vi "Autonomous Independent.vi"   [LabVIEW 2012]
doc: "This VI is called when autonomous begins, and will automatically be terminated when autonomous ends. You can carry out timed or sensor driven robot movement independently without needing to return to the caller."
uses:
  <vilib>/Rock Robotics/WPI/Relay/WPI_RelayValue.ctl
  <vilib>/Rock Robotics/WPI/DriverStation/DriverStationLCD/WPI_DriverStationLCDLCDLine.ctl
  <vilib>/Rock Robotics/WPI/CAN/Jaguar/SubVIs/WPI_CANJaguar_ControlMode.ctl
  <vilib>/Rock Robotics/WPI/CAN/Jaguar/SubVIs/WPI_CANJaguar_PositionReference.ctl
  <vilib>/Rock Robotics/WPI/CAN/Jaguar/SubVIs/WPI_CANJaguar_SpeedReference.ctl
  Robot Global Data.vi
types:
  T1 = typedef "WPI_DriverStationLCDLCDLine.ctl" = enum16{"Main - Line 1", "User - Line 2", "User - Line 3", "User - Line 4", "User - Line 5", "User - Line 6"}
  T2 = typedef "WPI_RelayValue.ctl" = enum16{"Off", "On", "Forward", "Reverse"}
  T3 = typedef "WPI_CANJaguar_ControlMode.ctl" = enum8{"Percent VBus", "Current", "Speed", "Position", "Voltage"}
  T4 = typedef "WPI_MotorControlDeviceRef.ctl" = cluster{"DeviceStatus":errorcluster, "Type":enum16{"PWM", "CAN"}, "PWM":cluster{"Digital Module":T5, "PWM Channel":T6, "DeadBand":T7}, "CAN":cluster{"Device Number":u8, "Control Mode":T3, "Semaphore":T8, "Max Vout":dbl}, "Invert":bool, "TransformRef":T9, "InvTransformRef":T9}
  T5 = typedef "FPGA_TypedefDigitalModule.ctl" = enum16{"Digital Module 1", "Digital Module 2"}
  T6 = typedef "FPGA_DIOPWMChannel.ctl" = enum8{"PWM 1", "PWM 2", "PWM 3", "PWM 4", "PWM 5", "PWM 6", "PWM 7", "PWM 8", "PWM 9", "PWM 10", "Invalid"}
  T7 = typedef "WPI_PWMDeadband.ctl" = cluster{"Name":string, "maxPositivePwm":i32, "minPositivePwm":i32, "centerPwm":i32, "maxNegativePwm":i32, "minNegativePwm":i32, "angularRange":u16}
  T8 = typedef "Semaphore RefNum" = refnum<k1>
  T9 = typedef "WPI_PWMTransform_ConPane.ctl" = refnum<vi>
  T10 = typedef "WPI_RelayDevRef.ctl" = cluster{"DevStatus":errorcluster, "Relay Channel":T11, "Digital Module":T5, "Relay Direction":T12}
  T11 = typedef "FPGA_DIORelayChannel.ctl" = enum8{"Relay 1", "Relay 2", "Relay 3", "Relay 4", "Relay 5", "Relay 6", "Relay 7", "Relay 8", "Invalid"}
  T12 = typedef "WPI_RelayDirection.ctl" = enum16{"Both directions", "Forward only", "Reverse only"}
  T13 = typedef "WPI_CANJaguar_PositionReference.ctl" = u8
  T14 = typedef "WPI_CANJaguar_SpeedReference.ctl" = u8
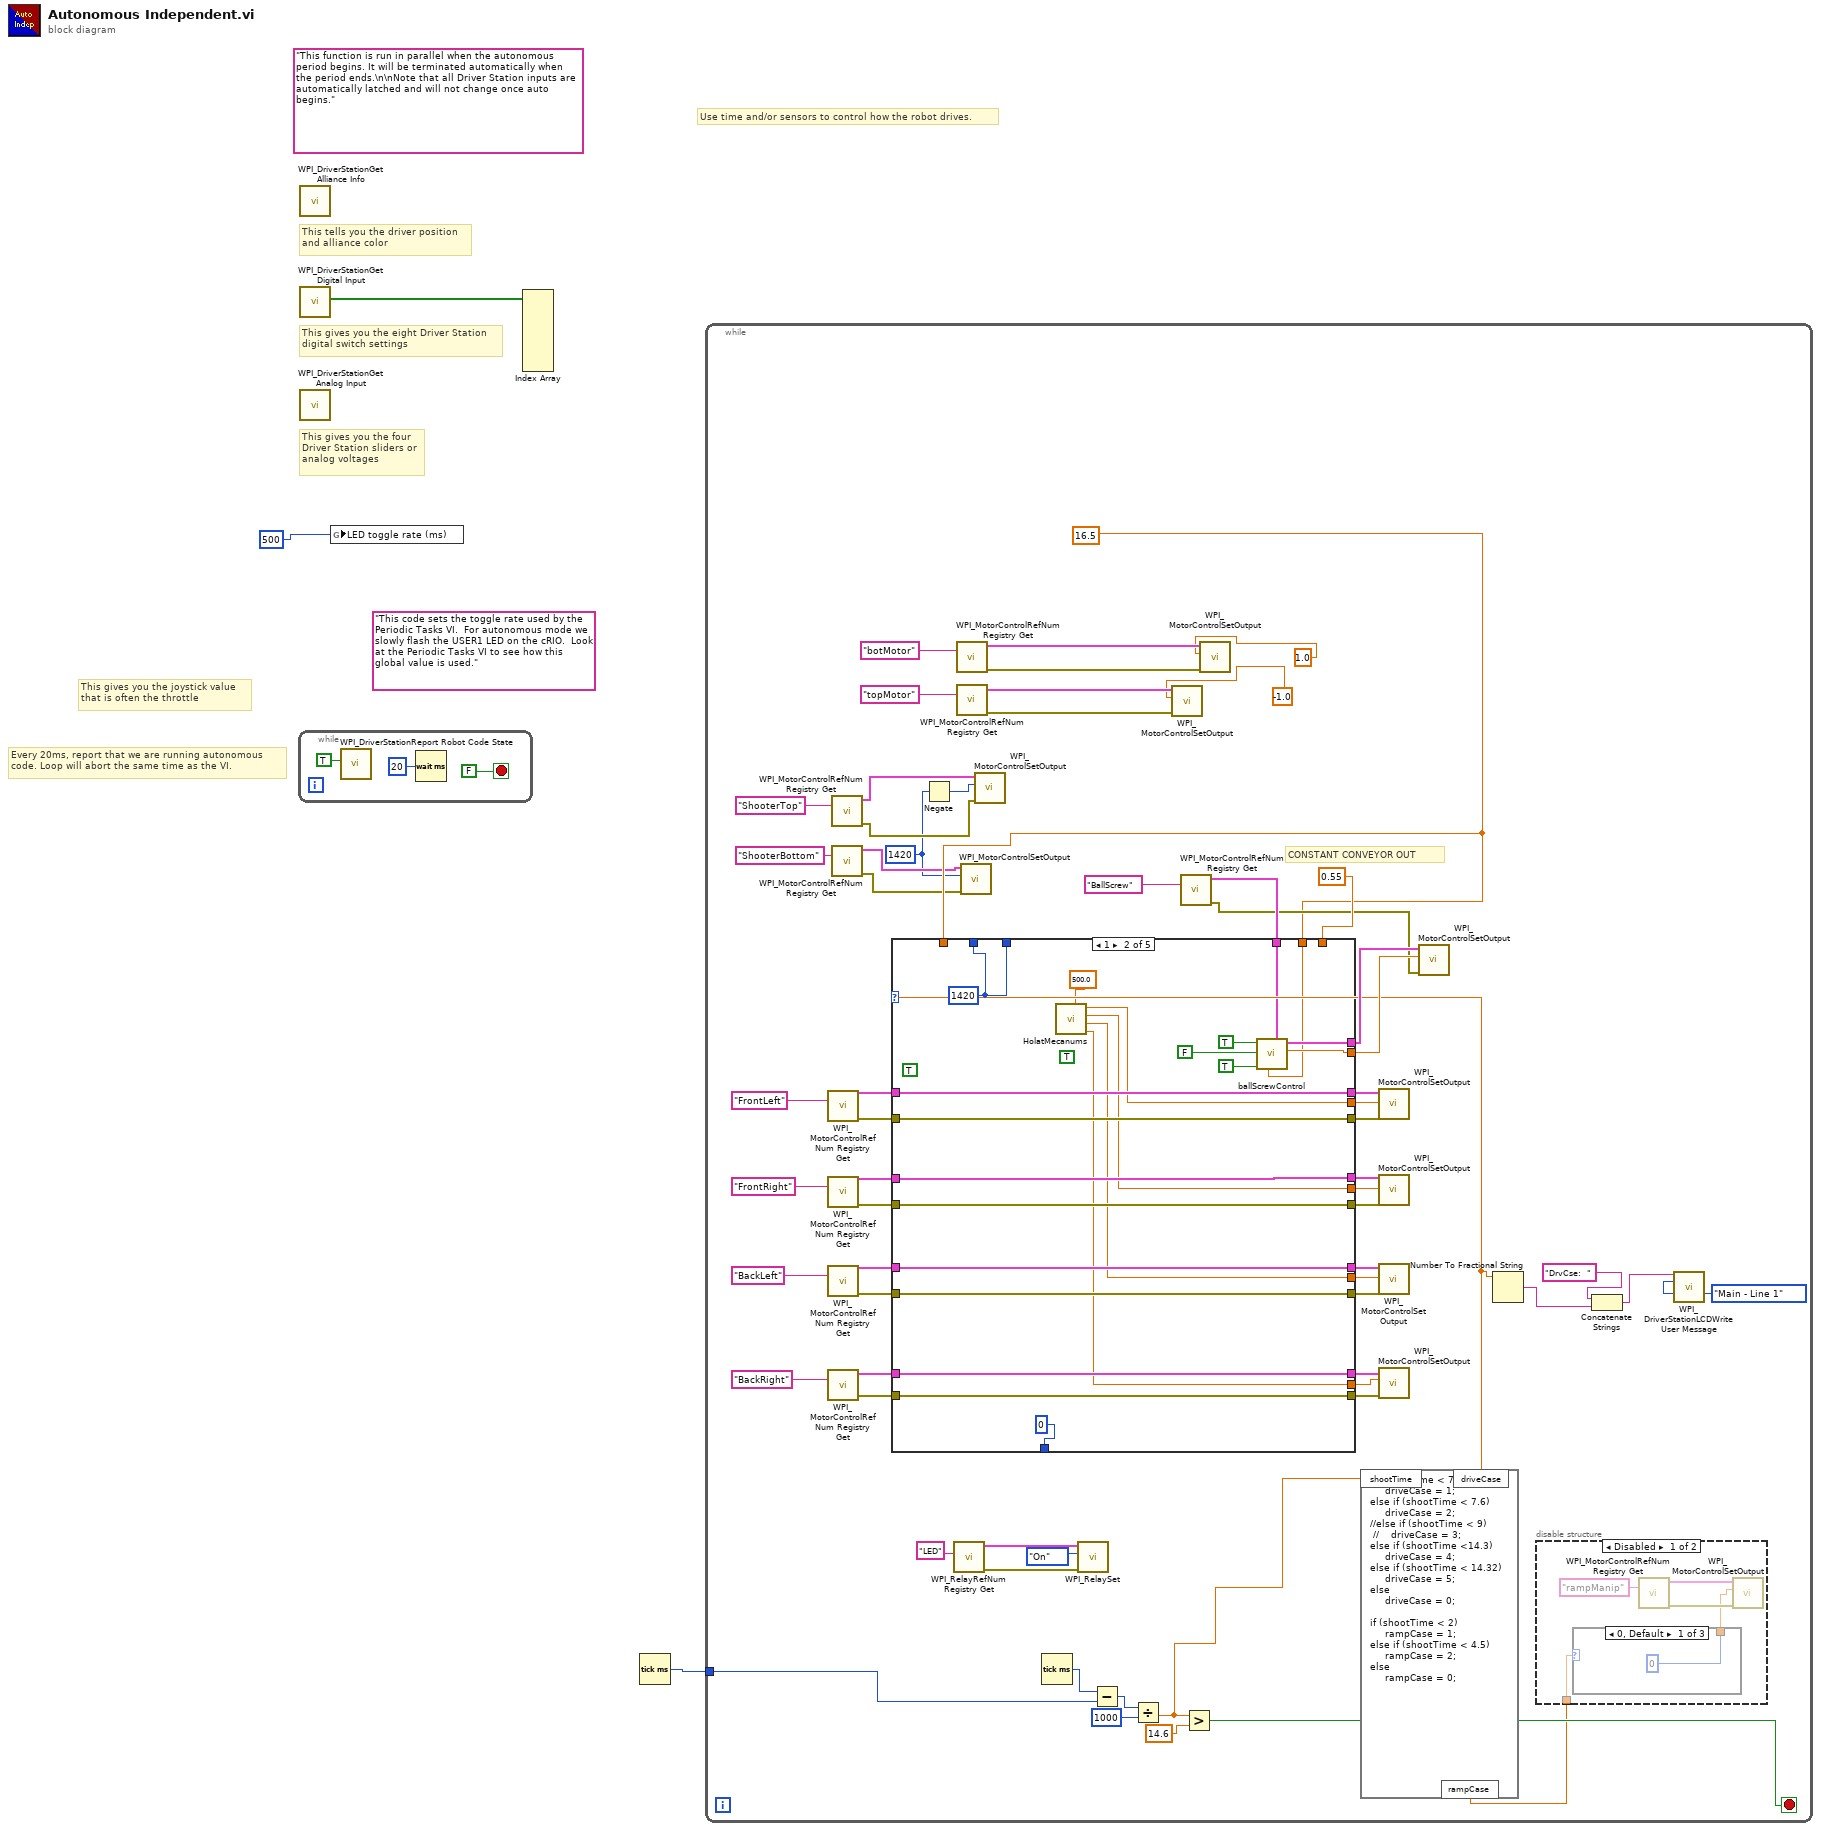
[diagram p0: block diagram]
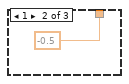
[diagram p2: hidden frame]
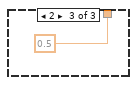
[diagram p3: hidden frame]
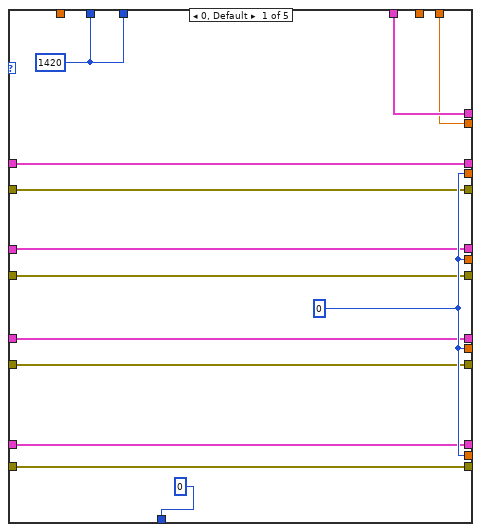
[diagram p5: hidden frame]
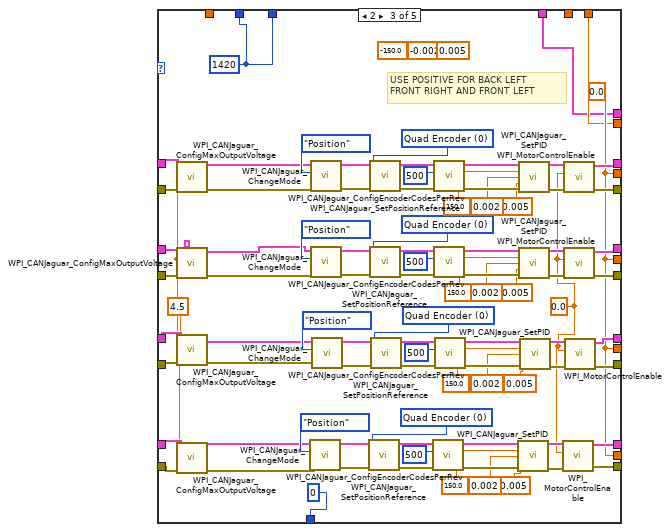
[diagram p6: hidden frame]
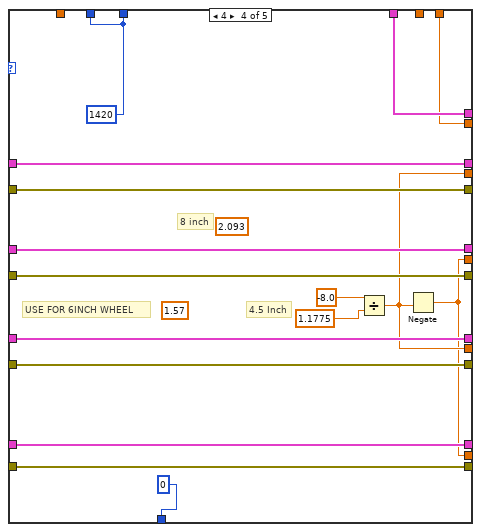
[diagram p7: hidden frame]
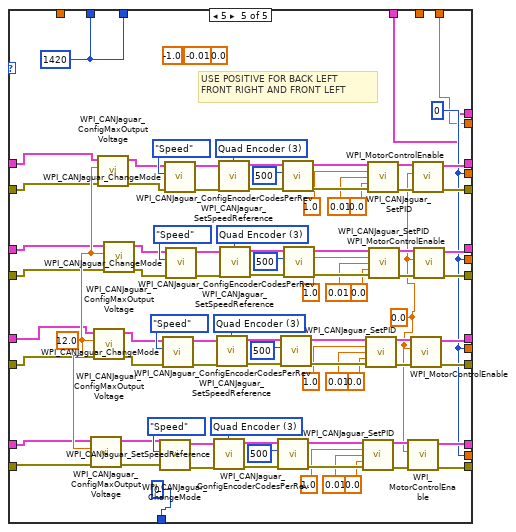
[diagram p8: hidden frame]
diagram:
  (unwired) "This code sets the toggle rate used by the Periodic Tasks VI.  For autonomous mode we slowly flash the USER1 LED on the cRIO.  Look at the Periodic Tasks VI to see how this global value is used."
  (unwired) "This function is run in parallel when the autonomous period begins. It will be terminated automatically when the period ends.\n\nNote that all Driver Station inputs are automatically latched and will not change once auto begins."
  # "Every 20ms, report that we are running autonomous\ncode. Loop will abort the same time as the VI."
  # "This gives you the joystick value\nthat is often the throttle"
  # "Use time and/or sensors to control how the robot drives."
  # "This tells you the driver position\nand alliance color"
  # "This gives you the eight Driver Station\ndigital switch settings"
  # "This gives you the four\nDriver Station sliders or\nanalog voltages"
  n1 = while {
    stop <- FALSE stop-if-true
    n2 = call <vilib>:"WPI_DriverStationReport Robot Code State.vi"("Autonomous"=TRUE) -> ()  [unwired: 10 in, 1 out]
    n3 = Wait (ms)(milliseconds to wait=u32 20) -> ()  [unwired: 1 out]
  }
  n4 = call <vilib>:"WPI_DriverStationGet Alliance Info.vi"() -> ()  [unwired: 12 out]
  n5 = call <vilib>:"WPI_DriverStationGet Digital Input.vi"() -> ("Driver Station Digital Input (1-8)"=w3:bool[])  [unwired: 11 out]
  n6 = call <vilib>:"WPI_DriverStationGet Analog Input.vi"() -> ()  [unwired: 12 out]
  n7 = global write "Robot Global Data.vi" "LED toggle rate (ms)"(u32 500 ("LED ms toggle rate")) -> ()
  n8 = Index Array(array=w3) -> ()  [unwired: 8 in, 8 out]
  n9 = Tick Count (ms)() -> (millisecond timer value=w2:u32)
  n10 = while {
    tunnel: w2 -> [w25]
    stop <- w26 stop-if-true
    w7 = 1420
    w13 = 16.5
    # "CONSTANT CONVEYOR OUT"
    n11 = call <vilib>:"WPI_MotorControlRefNum Registry Get.vi"("refnum name"="FrontLeft") -> ("error out"=w55:errorcluster, "MotorControlDevRef"=w54:T4)  [unwired: 9 in]
    n12 = call <vilib>:"WPI_MotorControlRefNum Registry Get.vi"("refnum name"="FrontRight") -> ("error out"=w57:errorcluster, "MotorControlDevRef"=w56:T4)  [unwired: 9 in]
    n13 = call <vilib>:"WPI_MotorControlRefNum Registry Get.vi"("refnum name"="BackLeft") -> ("error out"=w59:errorcluster, "MotorControlDevRef"=w58:T4)  [unwired: 9 in]
    n14 = call <vilib>:"WPI_MotorControlRefNum Registry Get.vi"("refnum name"="BackRight") -> ("error out"=w60:errorcluster, "MotorControlDevRef"=w61:T4)  [unwired: 9 in]
    n15 = call <vilib>:"WPI_MotorControlRefNum Registry Get.vi"("refnum name"="ShooterTop") -> ("error out"=w10:errorcluster, "MotorControlDevRef"=w11:T4)  [unwired: 9 in]
    n16 = call <vilib>:"WPI_MotorControlRefNum Registry Get.vi"("refnum name"="ShooterBottom") -> ("error out"=w8:errorcluster, "MotorControlDevRef"=w9:T4)  [unwired: 9 in]
    n17 = Negate(x=w7) -> (-x=w12:i32)
    n18 = call <vilib>:"WPI_RelayRefNum Registry Get.vi"("refnum name"="LED") -> ("error out"=w66:errorcluster, "RelayDevRef"=w67:T10)  [unwired: 9 in]
    n19 = call <vilib>:"WPI_MotorControlRefNum Registry Get.vi"("refnum name"="botMotor") -> ("error out"=w51:errorcluster, "MotorControlDevRef"=w52:T4)  [unwired: 9 in]
    n20 = call <vilib>:"WPI_MotorControlRefNum Registry Get.vi"("refnum name"="topMotor") -> ("error out"=w50:errorcluster, "MotorControlDevRef"=w69:T4)  [unwired: 9 in]
    n21 = call <vilib>:"WPI_MotorControlSetOutput.vi"("error in (no error)"=w8, "Output"=w7, "MotorControlDevRef"=w9) -> ()  [unwired: 6 in, 3 out]
    n22 = call <vilib>:"WPI_MotorControlSetOutput.vi"("error in (no error)"=w10, "Output"=w12, "MotorControlDevRef"=w11) -> ()  [unwired: 6 in, 3 out]
    n23 = Tick Count (ms)() -> (millisecond timer value=w46:u32)
    n24 = call <vilib>:"WPI_RelaySet.vi"("error in (no error)"=w66, "RelayValue"=WPI_RelayValue."On", "RelayDevRef"=w67) -> ()  [unwired: 7 in, 2 out]
    n25 = Subtract(x=w46, y=w25) -> (x-y=w45:u32)
    n26 = Divide(x=w45, y=u32 1000) -> (x/y=w27:dbl)
    n27 = call <vilib>:"WPI_MotorControlSetOutput.vi"("error in (no error)"=w50, "Output"=-1.0, "MotorControlDevRef"=w69) -> ()  [unwired: 6 in, 3 out]
    n28 = call <vilib>:"WPI_MotorControlRefNum Registry Get.vi"("refnum name"="BallScrew") -> ("error out"=w20:errorcluster, "MotorControlDevRef"=w24:T4)  [unwired: 9 in]
    n29 = Greater?(x=w27, y=14.6) -> (0:w26:bool)
    n30 = call <vilib>:"WPI_MotorControlSetOutput.vi"("error in (no error)"=w51, "Output"=1.0, "MotorControlDevRef"=w52) -> ()  [unwired: 6 in, 3 out]
    n31 = formula code="if (shootTime < 7.5)\n     driveCase = 1;\nelse if (shootTime < 7.6)\n     driveCase = 2;\n//else if (shootTime < 9)\n //    driveCase = 3;\nelse if (shootTime <14.3)\n     driveCase = 4;\nelse if (shootTime < 14.32)\n     driveCase = 5;\nelse\n     driveCase = 0;\n\nif (shootTime < 2)\n     rampCase = 1;\nelse if (shootTime < 4.5)\n     rampCase = 2;\nelse\n     rampCase = 0;"("shootTime"=w27) -> ("driveCase"=w14:dbl, "rampCase"=w19:dbl)
    n32 = case shown="1" w14 {
      tunnel: [w83 w112 w185 w216 w289] -> w36
      tunnel: w54 -> [w83 w112 w129 w216 w229]
      tunnel: [w85 w111 w170 w214 w273] -> w37
      tunnel: w56 -> [w85 w111 w134 w214 w231]
      tunnel: [w87 w110 w154 w212 w257] -> w38
      tunnel: w58 -> [w87 w110 w132 w212 w236]
      tunnel: [w89 w109 w138 w210 w241] -> w39
      tunnel: w61 -> [w89 w109 w128 w210 w234]
      tunnel: [w84 w108 w186 w215 w288] -> w32
      tunnel: w55 -> [w84 w108 w130 w215 w230]
      tunnel: [w86 w107 w169 w213 w272] -> w33
      tunnel: w57 -> [w86 w107 w133 w213 w232]
      tunnel: [w88 w106 w153 w211 w256] -> w34
      tunnel: w59 -> [w88 w106 w131 w211 w235]
      tunnel: [w90 w105 w137 w209 w240] -> w35
      tunnel: w60 -> [w90 w105 w127 w209 w233]
      tunnel: [w91 w104 w136 w206 w239] -> w31
      tunnel: [w91 w103 w136 w205 w239] -> w30
      tunnel: [w91 w102 w136 w206 w239] -> w29
      tunnel: [w91 w101 w136 w205 w239] -> w28
      tunnel: [0 0 0 0 0] -> _
      tunnel: w24 -> [w81 w96 w116 w204 w220]
      tunnel: [w81 w95 w116 w204 w220] -> w23
      tunnel: [w80 w94 w117 w203 w219] -> w22
      tunnel: w13 -> [_ w93 _ _ _]
      tunnel: 0.55 -> [w80 _ w117 w203 w219]
      tunnel: [w79 w92 w115 w202 w218] -> _
      tunnel: [w79 w92 w115 w202 w218] -> _
      tunnel: w13 -> [_ _ _ _ _]
      frame 0, Default {
        w79 = 1420
        w91 = 0
      }
      frame 1 {
        w92 = 1420
        (unwired) TRUE ("AutoTrack")
        (unwired) TRUE ("AUTO TRACK BUTTON")
        n33 = call "HolatMecanums.vi"("MaxOutput"=500.0) -> ("BackRight"=w101:dbl, "BackLeft"=w102:dbl, "FrontRight"=w103:dbl, "FrontLeft"=w104:dbl)  [unwired: 7 in]
        n34 = call "ballScrewControl.vi"("ballScrewMotorIN"=w96, "Distance"=w93, "autoTrackingButton"=TRUE, "ballScrewBotLimitSwitch"=FALSE, "ballScrewTopLimitSwitch"=TRUE) -> ("motorValueOutput"=w94:dbl, "ballScrewMotorOUT"=w95:T4)  [unwired: 5 in]
      }
      frame 2 {
        (unwired) 0.005 ("D")
        (unwired) -0.002 ("I")
        (unwired) -150.0 ("P")
        w114 = 0.0 ("Maximum Output Voltage")
        w115 = 1420
        w118 = 4.5 ("Maximum Output Voltage")
        w149 = T13 0 items=["Quad Encoder"=0, "Potentiometer"=1, "None"=255] ("Position Reference")
        w165 = T13 0 items=["Quad Encoder"=0, "Potentiometer"=1, "None"=255] ("Position Reference")
        w181 = T13 0 items=["Quad Encoder"=0, "Potentiometer"=1, "None"=255] ("Position Reference")
        w136 = 0.0 ("D")
        w197 = T13 0 items=["Quad Encoder"=0, "Potentiometer"=1, "None"=255] ("Position Reference")
        # "USE POSITIVE FOR BACK LEFT\nFRONT RIGHT AND FRONT LEFT"
        n35 = call <vilib>:"WPI_CANJaguar_ConfigMaxOutputVoltage.vi"("error in (no error)"=w130, "Maximum Output Voltage"=w118, "CAN Jaguar Ref"=w129) -> ("error out"=w120:errorcluster, "CAN Jaguar Ref Out"=w119:T4)  [unwired: 7 in]
        n36 = call <vilib>:"WPI_CANJaguar_ConfigMaxOutputVoltage.vi"("error in (no error)"=w133, "Maximum Output Voltage"=w118, "CAN Jaguar Ref"=w134) -> ("error out"=w122:errorcluster, "CAN Jaguar Ref Out"=w121:T4)  [unwired: 7 in]
        n37 = call <vilib>:"WPI_CANJaguar_ConfigMaxOutputVoltage.vi"("error in (no error)"=w131, "Maximum Output Voltage"=w118, "CAN Jaguar Ref"=w132) -> ("error out"=w124:errorcluster, "CAN Jaguar Ref Out"=w123:T4)  [unwired: 7 in]
        n38 = call <vilib>:"WPI_CANJaguar_ConfigMaxOutputVoltage.vi"("error in (no error)"=w127, "Maximum Output Voltage"=w118, "CAN Jaguar Ref"=w128) -> ("error out"=w126:errorcluster, "CAN Jaguar Ref Out"=w125:T4)  [unwired: 7 in]
        n39 = call <vilib>:"WPI_CANJaguar_ChangeMode.vi"("error in (no error)"=w126, "Control Mode"=WPI_CANJaguar_ControlMode."Position", "CAN Jaguar Ref"=w125) -> ("error out"=w151:errorcluster, "CAN Jaguar Ref Out"=w150:T4)  [unwired: 7 in]
        n40 = call <vilib>:"WPI_CANJaguar_ChangeMode.vi"("error in (no error)"=w120, "Control Mode"=WPI_CANJaguar_ControlMode."Position", "CAN Jaguar Ref"=w119) -> ("error out"=w199:errorcluster, "CAN Jaguar Ref Out"=w198:T4)  [unwired: 7 in]
        n41 = call <vilib>:"WPI_CANJaguar_ChangeMode.vi"("error in (no error)"=w122, "Control Mode"=WPI_CANJaguar_ControlMode."Position", "CAN Jaguar Ref"=w121) -> ("error out"=w183:errorcluster, "CAN Jaguar Ref Out"=w182:T4)  [unwired: 7 in]
        n42 = call <vilib>:"WPI_CANJaguar_ChangeMode.vi"("error in (no error)"=w124, "Control Mode"=WPI_CANJaguar_ControlMode."Position", "CAN Jaguar Ref"=w123) -> ("error out"=w167:errorcluster, "CAN Jaguar Ref Out"=w166:T4)  [unwired: 7 in]
        n43 = call <vilib>:"WPI_CANJaguar_SetPositionReference.vi"("error in (no error)"=w151, "Position Reference"=w149, "CAN Jaguar Ref"=w150) -> ("error out"=w148:errorcluster, "CAN Jaguar Ref Out"=w147:T4)  [unwired: 7 in]
        n44 = call <vilib>:"WPI_CANJaguar_SetPositionReference.vi"("error in (no error)"=w199, "Position Reference"=w197, "CAN Jaguar Ref"=w198) -> ("error out"=w196:errorcluster, "CAN Jaguar Ref Out"=w195:T4)  [unwired: 7 in]
        n45 = call <vilib>:"WPI_CANJaguar_SetPositionReference.vi"("error in (no error)"=w183, "Position Reference"=w181, "CAN Jaguar Ref"=w182) -> ("error out"=w180:errorcluster, "CAN Jaguar Ref Out"=w179:T4)  [unwired: 7 in]
        n46 = call <vilib>:"WPI_CANJaguar_SetPositionReference.vi"("error in (no error)"=w167, "Position Reference"=w165, "CAN Jaguar Ref"=w166) -> ("error out"=w164:errorcluster, "CAN Jaguar Ref Out"=w163:T4)  [unwired: 7 in]
        n47 = call <vilib>:"WPI_CANJaguar_ConfigEncoderCodesPerRev.vi"("error in (no error)"=w148, "Encoder Codes Per Rev"=u16 500, "CAN Jaguar Ref"=w147) -> ("error out"=w144:errorcluster, "CAN Jaguar Ref Out"=w145:T4)  [unwired: 7 in]
        n48 = call <vilib>:"WPI_CANJaguar_ConfigEncoderCodesPerRev.vi"("error in (no error)"=w196, "Encoder Codes Per Rev"=u16 500, "CAN Jaguar Ref"=w195) -> ("error out"=w192:errorcluster, "CAN Jaguar Ref Out"=w193:T4)  [unwired: 7 in]
        n49 = call <vilib>:"WPI_CANJaguar_ConfigEncoderCodesPerRev.vi"("error in (no error)"=w180, "Encoder Codes Per Rev"=u16 500, "CAN Jaguar Ref"=w179) -> ("error out"=w176:errorcluster, "CAN Jaguar Ref Out"=w177:T4)  [unwired: 7 in]
        n50 = call <vilib>:"WPI_CANJaguar_ConfigEncoderCodesPerRev.vi"("error in (no error)"=w164, "Encoder Codes Per Rev"=u16 500, "CAN Jaguar Ref"=w163) -> ("error out"=w160:errorcluster, "CAN Jaguar Ref Out"=w161:T4)  [unwired: 7 in]
        n51 = call <vilib>:"WPI_CANJaguar_SetPID.vi"("CAN Jaguar Ref"=w145, "P"=150.0, "I"=0.002, "D"=0.005, "error in (no error)"=w144) -> ("CAN Jaguar Ref Out"=w140:T4, "error out"=w139:errorcluster)  [unwired: 9 in]
        n52 = call <vilib>:"WPI_CANJaguar_SetPID.vi"("CAN Jaguar Ref"=w193, "P"=150.0, "I"=0.002, "D"=0.005, "error in (no error)"=w192) -> ("CAN Jaguar Ref Out"=w188:T4, "error out"=w187:errorcluster)  [unwired: 9 in]
        n53 = call <vilib>:"WPI_CANJaguar_SetPID.vi"("CAN Jaguar Ref"=w177, "P"=150.0, "I"=0.002, "D"=0.005, "error in (no error)"=w176) -> ("CAN Jaguar Ref Out"=w172:T4, "error out"=w171:errorcluster)  [unwired: 9 in]
        n54 = call <vilib>:"WPI_CANJaguar_SetPID.vi"("CAN Jaguar Ref"=w161, "P"=150.0, "I"=0.002, "D"=0.005, "error in (no error)"=w160) -> ("CAN Jaguar Ref Out"=w156:T4, "error out"=w155:errorcluster)  [unwired: 9 in]
        n55 = call <vilib>:"WPI_MotorControlEnable.vi"("error in (no error)"=w139, "Encoder Initial Position"=w114, "CAN Jaguar Ref"=w140) -> ("error out"=w137:errorcluster, "CAN Jaguar Ref Out"=w138:T4)  [unwired: 7 in]
        n56 = call <vilib>:"WPI_MotorControlEnable.vi"("error in (no error)"=w187, "Encoder Initial Position"=w114, "CAN Jaguar Ref"=w188) -> ("error out"=w186:errorcluster, "CAN Jaguar Ref Out"=w185:T4)  [unwired: 7 in]
        n57 = call <vilib>:"WPI_MotorControlEnable.vi"("error in (no error)"=w171, "Encoder Initial Position"=w114, "CAN Jaguar Ref"=w172) -> ("error out"=w169:errorcluster, "CAN Jaguar Ref Out"=w170:T4)  [unwired: 7 in]
        n58 = call <vilib>:"WPI_MotorControlEnable.vi"("error in (no error)"=w155, "Encoder Initial Position"=w114, "CAN Jaguar Ref"=w156) -> ("error out"=w153:errorcluster, "CAN Jaguar Ref Out"=w154:T4)  [unwired: 7 in]
      }
      frame 4 {
        (unwired) 1.57 ("D")
        (unwired) 2.093 ("D")
        w202 = 1420
        # "4.5 Inch"
        # "8 inch"
        # "USE FOR 6INCH WHEEL"
        n59 = Divide(x=-8.0, y=1.1775 ("D")) -> (x/y=w206:dbl)
        n60 = Negate(x=w206) -> (-x=w205:dbl)
      }
      frame 5 {
        (unwired) 0.0 ("D")
        (unwired) -0.01 ("I")
        (unwired) -1.0 ("P")
        w217 = 0.0 ("Maximum Output Voltage")
        w218 = 1420
        w237 = 12.0 ("Maximum Output Voltage")
        w239 = 0
        w252 = T14 3 items=["Encoder"=0, "Inv Encoder"=2, "Quad Encoder"=3, "None"=255] ("Speed Reference")
        w268 = T14 3 items=["Encoder"=0, "Inv Encoder"=2, "Quad Encoder"=3, "None"=255] ("Speed Reference")
        w284 = T14 3 items=["Encoder"=0, "Inv Encoder"=2, "Quad Encoder"=3, "None"=255] ("Speed Reference")
        w300 = T14 3 items=["Encoder"=0, "Inv Encoder"=2, "Quad Encoder"=3, "None"=255] ("Speed Reference")
        # "USE POSITIVE FOR BACK LEFT\nFRONT RIGHT AND FRONT LEFT"
        n61 = call <vilib>:"WPI_CANJaguar_ConfigMaxOutputVoltage.vi"("error in (no error)"=w233, "Maximum Output Voltage"=w237, "CAN Jaguar Ref"=w234) -> ("error out"=w221:errorcluster, "CAN Jaguar Ref Out"=w222:T4)  [unwired: 7 in]
        n62 = call <vilib>:"WPI_CANJaguar_ConfigMaxOutputVoltage.vi"("error in (no error)"=w235, "Maximum Output Voltage"=w237, "CAN Jaguar Ref"=w236) -> ("error out"=w223:errorcluster, "CAN Jaguar Ref Out"=w224:T4)  [unwired: 7 in]
        n63 = call <vilib>:"WPI_CANJaguar_ConfigMaxOutputVoltage.vi"("error in (no error)"=w230, "Maximum Output Voltage"=w237, "CAN Jaguar Ref"=w229) -> ("error out"=w227:errorcluster, "CAN Jaguar Ref Out"=w228:T4)  [unwired: 7 in]
        n64 = call <vilib>:"WPI_CANJaguar_ConfigMaxOutputVoltage.vi"("error in (no error)"=w232, "Maximum Output Voltage"=w237, "CAN Jaguar Ref"=w231) -> ("error out"=w225:errorcluster, "CAN Jaguar Ref Out"=w226:T4)  [unwired: 7 in]
        n65 = call <vilib>:"WPI_CANJaguar_ChangeMode.vi"("error in (no error)"=w221, "Control Mode"=WPI_CANJaguar_ControlMode."Speed", "CAN Jaguar Ref"=w222) -> ("error out"=w254:errorcluster, "CAN Jaguar Ref Out"=w253:T4)  [unwired: 7 in]
        n66 = call <vilib>:"WPI_CANJaguar_ChangeMode.vi"("error in (no error)"=w223, "Control Mode"=WPI_CANJaguar_ControlMode."Speed", "CAN Jaguar Ref"=w224) -> ("error out"=w270:errorcluster, "CAN Jaguar Ref Out"=w269:T4)  [unwired: 7 in]
        n67 = call <vilib>:"WPI_CANJaguar_ChangeMode.vi"("error in (no error)"=w227, "Control Mode"=WPI_CANJaguar_ControlMode."Speed", "CAN Jaguar Ref"=w228) -> ("error out"=w302:errorcluster, "CAN Jaguar Ref Out"=w301:T4)  [unwired: 7 in]
        n68 = call <vilib>:"WPI_CANJaguar_ChangeMode.vi"("error in (no error)"=w225, "Control Mode"=WPI_CANJaguar_ControlMode."Speed", "CAN Jaguar Ref"=w226) -> ("error out"=w286:errorcluster, "CAN Jaguar Ref Out"=w285:T4)  [unwired: 7 in]
        n69 = call <vilib>:"WPI_CANJaguar_SetSpeedReference.vi"("error in (no error)"=w254, "Speed Reference"=w252, "CAN Jaguar Ref"=w253) -> ("error out"=w245:errorcluster, "CAN Jaguar Ref Out"=w244:T4)  [unwired: 7 in]
        n70 = call <vilib>:"WPI_CANJaguar_SetSpeedReference.vi"("error in (no error)"=w270, "Speed Reference"=w268, "CAN Jaguar Ref"=w269) -> ("error out"=w261:errorcluster, "CAN Jaguar Ref Out"=w260:T4)  [unwired: 7 in]
        n71 = call <vilib>:"WPI_CANJaguar_SetSpeedReference.vi"("error in (no error)"=w302, "Speed Reference"=w300, "CAN Jaguar Ref"=w301) -> ("error out"=w293:errorcluster, "CAN Jaguar Ref Out"=w292:T4)  [unwired: 7 in]
        n72 = call <vilib>:"WPI_CANJaguar_SetSpeedReference.vi"("error in (no error)"=w286, "Speed Reference"=w284, "CAN Jaguar Ref"=w285) -> ("error out"=w277:errorcluster, "CAN Jaguar Ref Out"=w276:T4)  [unwired: 7 in]
        n73 = call <vilib>:"WPI_CANJaguar_ConfigEncoderCodesPerRev.vi"("error in (no error)"=w245, "Encoder Codes Per Rev"=u16 500, "CAN Jaguar Ref"=w244) -> ("error out"=w250:errorcluster, "CAN Jaguar Ref Out"=w243:T4)  [unwired: 7 in]
        n74 = call <vilib>:"WPI_CANJaguar_ConfigEncoderCodesPerRev.vi"("error in (no error)"=w261, "Encoder Codes Per Rev"=u16 500, "CAN Jaguar Ref"=w260) -> ("error out"=w266:errorcluster, "CAN Jaguar Ref Out"=w259:T4)  [unwired: 7 in]
        n75 = call <vilib>:"WPI_CANJaguar_ConfigEncoderCodesPerRev.vi"("error in (no error)"=w293, "Encoder Codes Per Rev"=u16 500, "CAN Jaguar Ref"=w292) -> ("error out"=w298:errorcluster, "CAN Jaguar Ref Out"=w291:T4)  [unwired: 7 in]
        n76 = call <vilib>:"WPI_CANJaguar_ConfigEncoderCodesPerRev.vi"("error in (no error)"=w277, "Encoder Codes Per Rev"=u16 500, "CAN Jaguar Ref"=w276) -> ("error out"=w282:errorcluster, "CAN Jaguar Ref Out"=w275:T4)  [unwired: 7 in]
        n77 = call <vilib>:"WPI_CANJaguar_SetPID.vi"("CAN Jaguar Ref"=w243, "P"=1.0, "I"=0.01, "D"=0.0, "error in (no error)"=w250) -> ("CAN Jaguar Ref Out"=w242:T4, "error out"=w246:errorcluster)  [unwired: 9 in]
        n78 = call <vilib>:"WPI_CANJaguar_SetPID.vi"("CAN Jaguar Ref"=w259, "P"=1.0, "I"=0.01, "D"=0.0, "error in (no error)"=w266) -> ("CAN Jaguar Ref Out"=w258:T4, "error out"=w262:errorcluster)  [unwired: 9 in]
        n79 = call <vilib>:"WPI_CANJaguar_SetPID.vi"("CAN Jaguar Ref"=w291, "P"=1.0, "I"=0.01, "D"=0.0, "error in (no error)"=w298) -> ("CAN Jaguar Ref Out"=w290:T4, "error out"=w294:errorcluster)  [unwired: 9 in]
        n80 = call <vilib>:"WPI_CANJaguar_SetPID.vi"("CAN Jaguar Ref"=w275, "P"=1.0, "I"=0.01, "D"=0.0, "error in (no error)"=w282) -> ("CAN Jaguar Ref Out"=w274:T4, "error out"=w278:errorcluster)  [unwired: 9 in]
        n81 = call <vilib>:"WPI_MotorControlEnable.vi"("error in (no error)"=w246, "Encoder Initial Position"=w217, "CAN Jaguar Ref"=w242) -> ("error out"=w240:errorcluster, "CAN Jaguar Ref Out"=w241:T4)  [unwired: 7 in]
        n82 = call <vilib>:"WPI_MotorControlEnable.vi"("error in (no error)"=w262, "Encoder Initial Position"=w217, "CAN Jaguar Ref"=w258) -> ("error out"=w256:errorcluster, "CAN Jaguar Ref Out"=w257:T4)  [unwired: 7 in]
        n83 = call <vilib>:"WPI_MotorControlEnable.vi"("error in (no error)"=w294, "Encoder Initial Position"=w217, "CAN Jaguar Ref"=w290) -> ("error out"=w288:errorcluster, "CAN Jaguar Ref Out"=w289:T4)  [unwired: 7 in]
        n84 = call <vilib>:"WPI_MotorControlEnable.vi"("error in (no error)"=w278, "Encoder Initial Position"=w217, "CAN Jaguar Ref"=w274) -> ("error out"=w272:errorcluster, "CAN Jaguar Ref Out"=w273:T4)  [unwired: 7 in]
      }
    }
    n85 = call <vilib>:"WPI_MotorControlSetOutput.vi"("error in (no error)"=w32, "Output"=w31, "MotorControlDevRef"=w36) -> ()  [unwired: 6 in, 3 out]
    n86 = call <vilib>:"WPI_MotorControlSetOutput.vi"("error in (no error)"=w33, "Output"=w30, "MotorControlDevRef"=w37) -> ()  [unwired: 6 in, 3 out]
    n87 = call <vilib>:"WPI_MotorControlSetOutput.vi"("error in (no error)"=w34, "Output"=w29, "MotorControlDevRef"=w38) -> ()  [unwired: 6 in, 3 out]
    n88 = call <vilib>:"WPI_MotorControlSetOutput.vi"("error in (no error)"=w35, "Output"=w28, "MotorControlDevRef"=w39) -> ()  [unwired: 6 in, 3 out]
    n89 = call <vilib>:"WPI_MotorControlSetOutput.vi"("error in (no error)"=w20, "Output"=w22, "MotorControlDevRef"=w23) -> ()  [unwired: 6 in, 3 out]
    n90 = Number To Fractional String(number=w14) -> (F-format string=w16:string)  [unwired: 3 in]
    n91 = disable-structure shown="Disabled" {
      disable-tunnel: w19 -> [w72 _]
      frame Disabled {
        n92 = case shown="0, Default" w72 {
          tunnel: [0 -0.5 0.5] -> w71
          frame 0, Default {
          }
          frame 1 {
          }
          frame 2 {
          }
        }
        n93 = call <vilib>:"WPI_MotorControlRefNum Registry Get.vi"("refnum name"="rampManip") -> ("error out"=w73:errorcluster, "MotorControlDevRef"=w74:T4)  [unwired: 9 in]
        n94 = call <vilib>:"WPI_MotorControlSetOutput.vi"("error in (no error)"=w73, "Output"=w71, "MotorControlDevRef"=w74) -> ()  [unwired: 6 in, 3 out]
      }
      frame Enabled {
      }
    }
    n95 = Concatenate Strings("DrvCse:  " ("line text"), w16) -> (w15:string)
    n96 = call <vilib>:"WPI_DriverStationLCDWrite User Message.vi"("line text"=w15, "line"=WPI_DriverStationLCDLCDLine."Main - Line 1") -> ()  [unwired: 13 in, 1 out]
  }
